vi "File.Copy_Move File or Dir to a Dir.vi"(8 "error in":errorcluster, 9 "Copy(F)/Move(T)":bool, 10 "Destination":path, 11 "Source":path) -> (0 "error out":errorcluster, 3 "Dest Dup":path)   [LabVIEW 2024]
uses:
  <vilib>/KATE/Files/File Utils.lvlib
panel:
  in  "Error if Source Does not Exist":bool
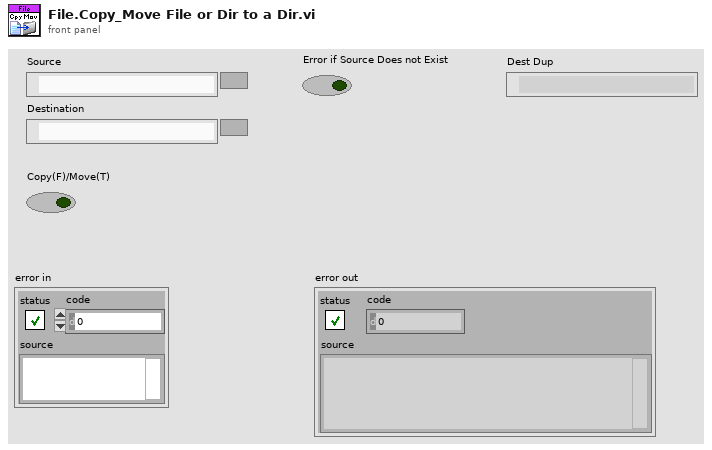
[diagram p1: front panel]
types:
  T1 = cluster{"IsDir":bool, "Exists":bool, "Path":path}
  T2 = cluster{"Source":cluster{"IsDir":bool, "Exists":bool, "Path":path}, "Dest":cluster{"IsDir":bool, "Exists":bool, "Path":path}}
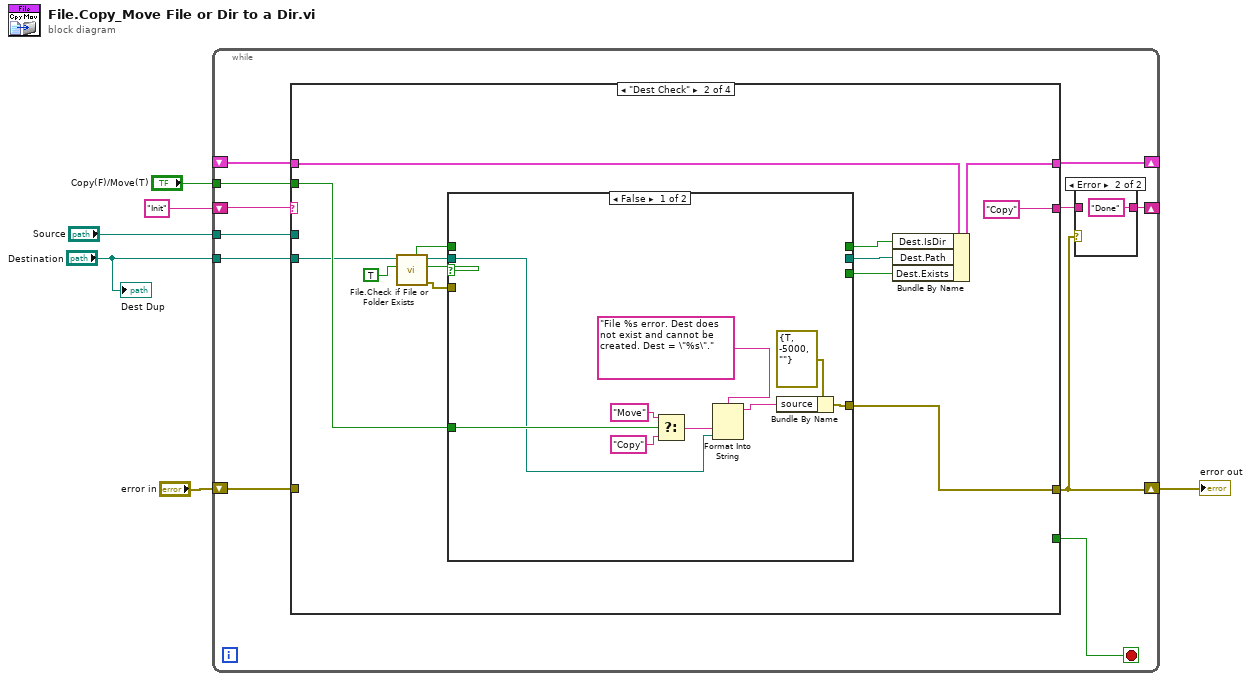
[diagram p0: block diagram]
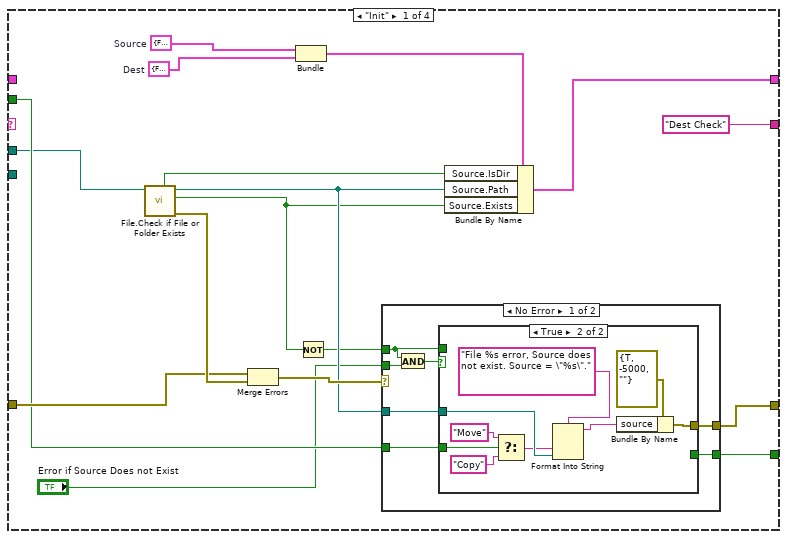
[diagram p3: hidden frame]
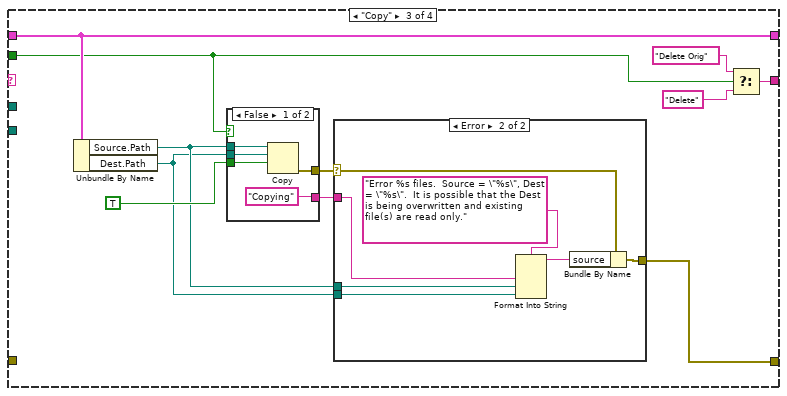
[diagram p7: hidden frame]
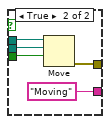
[diagram p8: hidden frame]
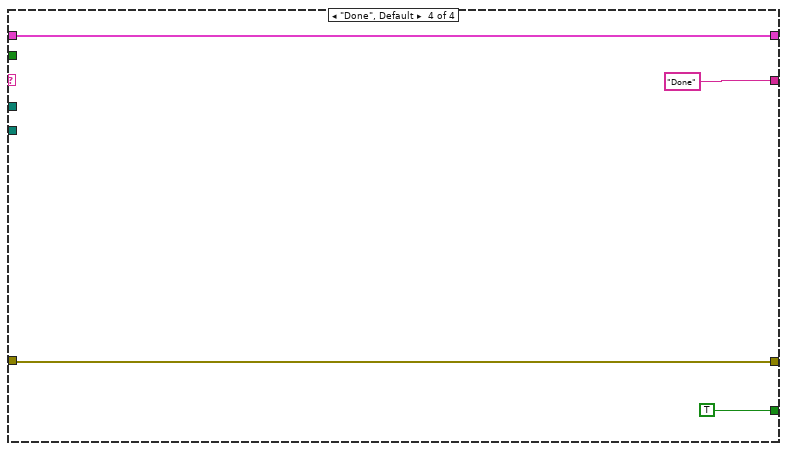
[diagram p10: hidden frame]
diagram:
  n1 = while {
    shift-right: [w10] -> _
    shift-left: "Init" -> [w17]
    shift-right: [w15] -> _
    shift-left: _ -> [w16]
    shift-right: [w12] -> w4
    shift-left: "error in" -> [w13]
    tunnel: "Copy(F)/Move(T)" -> [w9]
    tunnel: "Source" -> [w8]
    tunnel: "Destination" -> [w7]
    stop <- w11 stop-if-true
    n2 = case shown="\"Dest Check\"" w17 {
      tunnel: w16 -> [_ w67 w90 w111]
      tunnel: [w22 w66 w90 w111] -> w15
      tunnel: ["Dest Check" "Copy" w85 "Done"] -> w14
      tunnel: [w30 w57 w86 w109] -> w12
      tunnel: w13 -> [w29 _ _ w109]
      tunnel: [w23 _ _ TRUE] -> w11
      tunnel: w9 -> [w27 w56 w82 _]
      tunnel: w8 -> [w20 _ _ _]
      tunnel: w7 -> [_ w55 _ _]
      frame "Init" {
        w35 = T1 {"IsDir"=FALSE, "Exists"=FALSE, "Path"=path ""}  # Dest
        w36 = T1 {"IsDir"=FALSE, "Exists"=FALSE, "Path"=path ""}  # Source
        n3 = call <vilib>:"File.Check if File or Folder Exists.vi"("Path"=w20) -> ("error out"=w32:errorcluster, "Exists"=w26:bool, "Dup Path"=w28:path, "IsDir"=w33:bool)  [unwired: 6 in, 1 out]
        n4 = Merge Errors(w29, w32) -> (w31:errorcluster)
        n5 = Bundle("Source"=w36, "Dest"=w35) -> (w21:T2)  [unwired: 1 in]
        n6 = Not(x=w26) -> (.not. x?=w25:bool)
        n7 = case shown="No Error" w31 {
          selector: w31 -> [_ w54]
          tunnel: [w43 w54] -> w30
          tunnel: w28 -> [w42 _]
          tunnel: w27 -> [w41 _]
          tunnel: w25 -> [w37 _]
          tunnel: "Error if Source Does not Exist" -> [w39 _]
          tunnel: [w38 _] -> w23
          frame No Error {
            n8 = And(x=w37, y=w39) -> (x .and. y?=w40:bool)
            n9 = case shown="True" w40 {
              tunnel: [_ w52] -> w43
              tunnel: w42 -> [_ w49]
              tunnel: w41 -> [_ w47]
              tunnel: [w44 _] -> w38
              tunnel: w37 -> [w44 _]
              frame False {
              }
              frame True {
                n10 = Select(t="Move", s=w47, f="Copy") -> (s? t:f=w48:string)
                n11 = Format Into String(format string="File %s error, Source does not exist. Source = \"%s\".", w48, w49) -> (resulting string=w50:string)  [unwired: 2 in, 1 out]
                n12 = Bundle By Name(cluster=errorcluster {"status"=TRUE, "code"=-5000, "source"=""} ("error constant"), "source"=w50) -> (w52:errorcluster)
              }
            }
          }
          frame Error {
          }
        }
        n13 = Bundle By Name(cluster=w21, "Source.IsDir"=w33, "Source.Path"=w28, "Source.Exists"=w26) -> (w22:T2)
      }
      frame "Dest Check" {
        n14 = call <vilib>:"File.Check if File or Folder Exists.vi"("Create Dir if does not Exist"=TRUE, "Path"=w55) -> ("error out"=w63:errorcluster, "Exists"=w64:bool, "Dup Path"=w62:path, "IsDir"=w61:bool)  [unwired: 5 in, 1 out]
        n15 = case shown="False" w64 {
          selector: w64 -> [_ w79]
          tunnel: w63 -> [_ _]
          tunnel: w62 -> [w69 w78]
          tunnel: w61 -> [_ w80]
          tunnel: [_ w80] -> w60
          tunnel: [_ w78] -> w59
          tunnel: [_ w79] -> w58
          tunnel: [w71 _] -> w57
          tunnel: w56 -> [w70 _]
          frame False {
            n16 = Select(t="Move", s=w70, f="Copy") -> (s? t:f=w74:string)
            n17 = Format Into String(format string="File %s error. Dest does not exist and cannot be created. Dest = \"%s\".", w74, w69) -> (resulting string=w75:string)  [unwired: 2 in, 1 out]
            n18 = Bundle By Name(cluster=errorcluster {"status"=TRUE, "code"=-5000, "source"=""} ("error constant"), "source"=w75) -> (w71:errorcluster)
          }
          frame True {
          }
        }
        n19 = Bundle By Name(cluster=w67, "Dest.IsDir"=w60, "Dest.Path"=w59, "Dest.Exists"=w58) -> (w66:T2)
      }
      frame "Copy" {
        n20 = Unbundle By Name(w90) -> ("Source.Path"=w89:path, "Dest.Path"=w88:path)
        n21 = case shown="False" w82 {
          tunnel: TRUE ("overwrite (F)") -> [w96 w98]
          tunnel: w89 -> [w95 w100]
          tunnel: w88 -> [w94 w99]
          tunnel: [w93 w101] -> w87
          tunnel: ["Copying" "Moving"] -> w81
          frame False {
            n22 = Copy(9:w96, 10:w94, 11:w95) -> (0:w93:errorcluster)  [unwired: 2 in, 2 out]
          }
          frame True {
            n23 = Move(source path=w100, 9:w98, 10:w99) -> (error out=w101:errorcluster)  [unwired: 2 in, 2 out]
          }
        }
        n24 = case shown="Error" w87 {
          selector: w87 -> [_ w104]
          tunnel: w89 -> [_ w106]
          tunnel: w88 -> [_ w105]
          tunnel: [_ w103] -> w86
          tunnel: w81 -> [_ w102]
          frame No Error {
          }
          frame Error {
            n25 = Format Into String(format string="Error %s files.  Source = \"%s\", Dest = \"%s\".  It is possible that the Dest is being overwritten and existing file(s) are read only.", w102, w106, w105) -> (resulting string=w107:string)  [unwired: 2 in, 1 out]
            n26 = Bundle By Name(cluster=w104, "source"=w107) -> (w103:errorcluster)
          }
        }
        n27 = Select(t="Delete Orig", s=w82, f="Delete") -> (s? t:f=w85:string)
      }
      frame "Done", Default {
      }
    }
    n28 = case shown="Error" w12 {
      tunnel: w14 -> [w18 _]
      tunnel: [w18 "Done"] -> w10
      frame No Error {
      }
      frame Error {
      }
    }
  }
  "error out" <- w4
  "Dest Dup" <- "Destination"
